vi "Save Packets.vi"(8 "error in (no error)":errorcluster, 10 "Save Packets":bool, 11 "Packets in":string[](array[string])) -> (0 "error out":errorcluster)   [LabVIEW 2017]
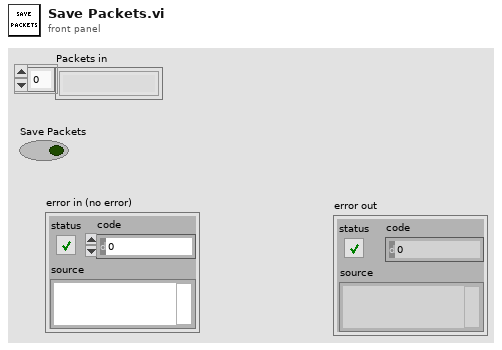
[diagram p1: front panel]
types:
  T1 = enum16{"open", "replace", "create", "open or create", "replace or create", "replace or create with confirmation"}
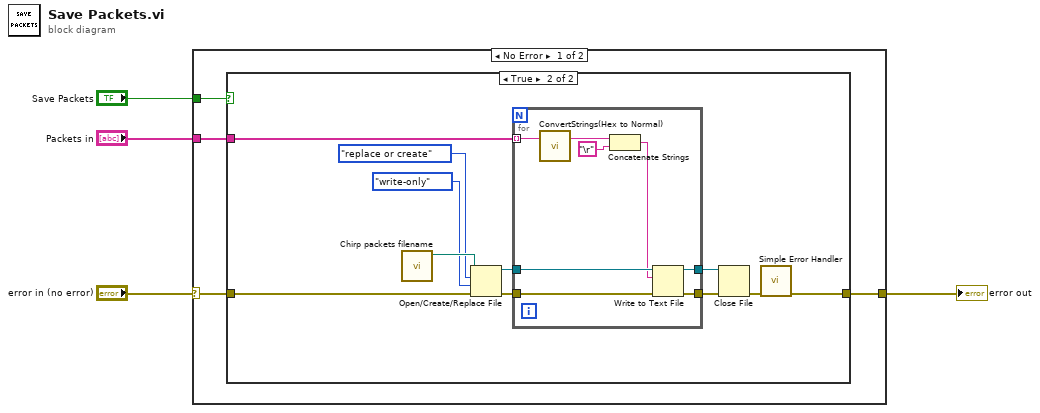
[diagram p0: block diagram]
diagram:
  n1 = case shown="No Error" "error in (no error)" {
    selector: "error in (no error)" -> [w5 w29]
    tunnel: "Packets in" -> [w8 _]
    tunnel: "Save Packets" -> [w7 _]
    tunnel: [w6 w29] -> w2
    frame No Error {
      n2 = case shown="True" w7 {
        tunnel: w8 -> [_ w20]
        tunnel: w5 -> [w9 w17]
        tunnel: [w9 w19] -> w6
        frame False {
        }
        frame True {
          n3 = call "Chirp packets filename.vi"() -> ("Packets file path"=w18:path)  [unwired: 10 in, 1 out]
          n4 = Open/Create/Replace File(file path (use dialog)=w18, error in=w17, operation (0:open)=T1."replace or create", access (0:read/write)=enum16{"read/write", "read-only", "write-only"}."write-only") -> (refnum out=w12:refnum<file>, error out=w13:errorcluster)  [unwired: 3 out]
          n5 = for {
            tunnel: w20 -> [w24] mode=indexing
            tunnel: w13 -> [w28]
            tunnel: w12 -> [w27]
            tunnel: [w26] -> w11
            tunnel: [w25] -> w10
            n6 = call "ConvertStrings(Hex to Normal).vi"("Hex String"=w24) -> ("Normal String"=w22:string)  [unwired: 2 in]
            n7 = Concatenate Strings(w22, "\r") -> (w23:string)
            n8 = Write to Text File(file (use dialog)=w27, text=w23, error in=w28) -> (refnum out=w26:refnum<file>, error out=w25:errorcluster)  [unwired: 1 in, 1 out]
          }
          n9 = Close File(refnum=w11, error in=w10) -> (error out=w14:errorcluster)  [unwired: 1 out]
          n10 = call <vilib>:"Simple Error Handler.vi"("error in (no error)"=w14) -> ("error out"=w19:errorcluster)  [unwired: 2 in, 6 out]
        }
      }
    }
    frame Error {
    }
  }
  "error out" <- w2
